vi "Bode Magnitude Plot.vi"() -> ()   [LabVIEW 2015]
uses:
  <vilib>/Analysis/NI_AALPro.lvlib
panel:
  out "x*y":dbl
  out "AC estimate (Vrms)":dbl format="%0.2f"
  out "x+y":i32
  out "XY Graph":cluster{dbl[], dbl[]}(graph)
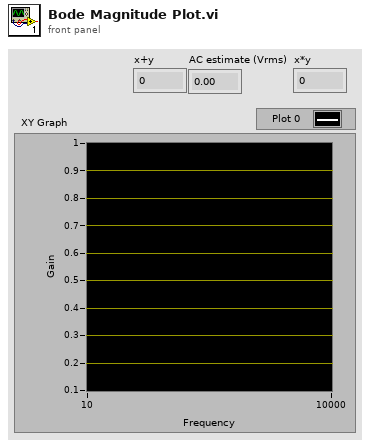
[diagram p1: front panel]
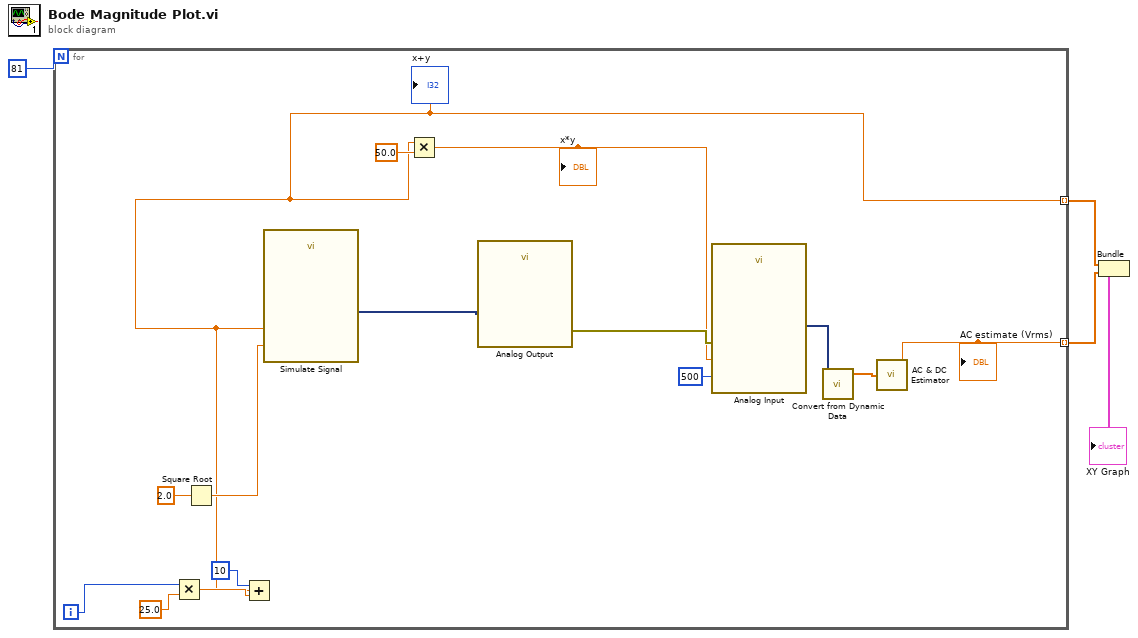
[diagram p0: block diagram]
diagram:
  n1 = for {
    N: 81 ("Numeric") -> [_]
    tunnel: [w6] -> w4 mode=indexing
    tunnel: [w10] -> w3 mode=indexing
    i -> [w5]
    n2 = Multiply(x=w5, y=25.0) -> (x*y=w8:dbl)
    n3 = Square Root(x=2.0) -> (sqrt(x)=w16:dbl)
    n4 = Add(x=10, y=w8) -> (x+y=w6:dbl)
    "x+y" <- w6
    n5 = call "Simulate Signal"("Frequency"=w6, "Amplitude"=w16) -> ("Sine"=w19:dynamicdata)  [unwired: 12 in, 1 out]
    n6 = Multiply(x=w6, y=50.0) -> (x*y=w14:dbl)
    "x*y" <- w14
    n7 = call "Analog Output"("data"=w19) -> ("error out"=w18:errorcluster)  [unwired: 16 in, 2 out]
    n8 = call "Analog Input"("rate"=w14, "number of samples"=500, "error in"=w18) -> ("data"=w12:dynamicdata)  [unwired: 14 in, 2 out]
    n9 = call "Convert from Dynamic Data"("Dynamic Data Type"=w12) -> ("Array"=w11:dbl[])  [unwired: 3 in]
    n10 = call <vilib>:"AC & DC Estimator.vi"("Signal (V)"=w11) -> ("AC estimate (Vrms)"=w10:dbl)  [unwired: 1 out]
    "AC estimate (Vrms)" <- w10
  }
  n11 = Bundle(w4, w3) -> (→"XY Graph":cluster{dbl[], dbl[]})  [unwired: 1 in]
